vi "MccHat_format_data.vi"(8 "readings":cluster{i32, i32, dbl}[](array[cluster]), 11 "time":timestamp) -> (3 "waveform_array_A":waveform(dbl)[](array[waveform])=[{"t0"=timestamp(0 s since 1904-01-01), "dt"=1.0, "Y"=[]}, {"t0"=timestamp(3732035173.078092 s since 1904-01-01), "dt"=1.0, "Y"=[302.8589782714844], "attributes"=variant("NI_ChannelName"=variant(string "T1"))}])   [LabVIEW 2019]
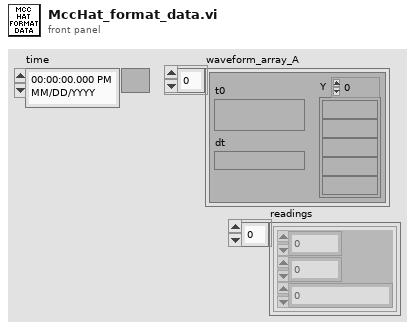
[diagram p1: front panel]
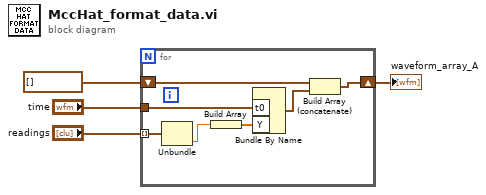
[diagram p0: block diagram]
diagram:
  n1 = for {
    tunnel: "time" -> [w9]
    shift-right: [w8] -> w4
    shift-left: waveform(dbl)[] [] -> [w11]
    tunnel: "readings" -> [w6] mode=indexing
    n2 = Unbundle(w6) -> (w5:dbl)  [unwired: 2 out]
    n3 = Build Array(w5) -> (w10:dbl[])
    n4 = Bundle By Name("t0"=w9, "Y"=w10) -> (w7:waveform(dbl))  [unwired: 1 in]
    n5 = Build Array (concatenate)(w11, w7) -> (w8:waveform(dbl)[])
  }
  "waveform_array_A" <- w4
